vi "InitClassQueue.vi"(8 "ErrorIn(No Error)":errorcluster caption="entrée d'erreur (pas d'erreur)", 10 "Session":string, 11 "BaseDevice.lvclass":refnum<class "BaseDevice.lvclass">) -> (0 "sortie d'erreur":errorcluster, 1 "InstrClassQ":refnum<queue>, 2 "InstrClassEvent":refnum<user-event>, 3 "BaseDevice.lvclass Out":refnum<class "BaseDevice.lvclass">)   [LabVIEW 2019, in "BaseDevice.lvclass"]
uses:
  BaseDevice.lvclass
  BaseDevice.lvclass/BaseDevice.ctl
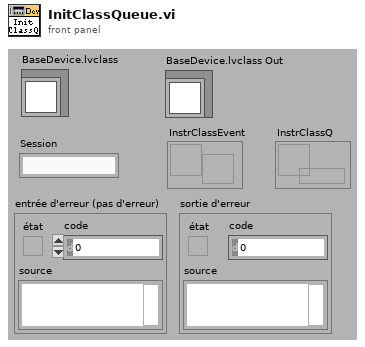
[diagram p1: front panel]
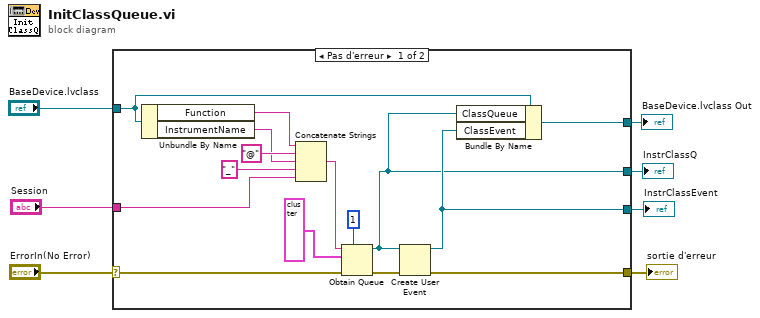
[diagram p0: block diagram]
diagram:
  n1 = case shown="Pas d'erreur" "ErrorIn(No Error)" {
    selector: "ErrorIn(No Error)" -> [w18 w24]
    tunnel: [w19 w24] -> w7
    tunnel: "BaseDevice.lvclass" -> [w17 w23]
    tunnel: [w16 w23] -> w4
    tunnel: "Session" -> [w10 _]
    tunnel: [w9 _] -> w2
    tunnel: [w8 _] -> w1
    frame No Error {
      n2 = Unbundle By Name(w17) -> ("Function"=w14:string, "InstrumentName"=w13:string)
      n3 = Concatenate Strings(w14, "@" ("chaîne"), w13, "_" ("chaîne"), w10) -> (w12:string)
      n4 = Obtain Queue(max queue size (-1, unlimited)=1 ("taille max de la file d'attente (-1, non limitée)"), name (unnamed)=w12, element data type=cluster{"Message":string, "Data":variant, i32} {"Message"="", "Data"=variant, 0} ("ClassQueue"), error in (no error)=w18) -> (queue out=w8:refnum<queue>, error out=w20:errorcluster)  [unwired: 1 in, 1 out]
      n5 = Create User Event(user event datatype=w8, error in=w20) -> (user event=w9:refnum<user-event>, error out=w19:errorcluster)
      n6 = Bundle By Name(cluster=w17, "ClassQueue"=w8, "ClassEvent"=w9) -> (w16:refnum<class "BaseDevice.lvclass">)
    }
    frame Error {
    }
  }
  "sortie d'erreur" <- w7
  "BaseDevice.lvclass Out" <- w4
  "InstrClassEvent" <- w2
  "InstrClassQ" <- w1
